vi "NLR3.vi"(8 "X4":dbl, 9 "X3":dbl, 10 "X2":dbl, 11 "X1":dbl) -> (2 "s? t:f":dbl)   [LabVIEW 2013]
uses:
  <vilib>/express/express arith-compare/Formula/XNode/ExpressFormulaBlockNode.xnode
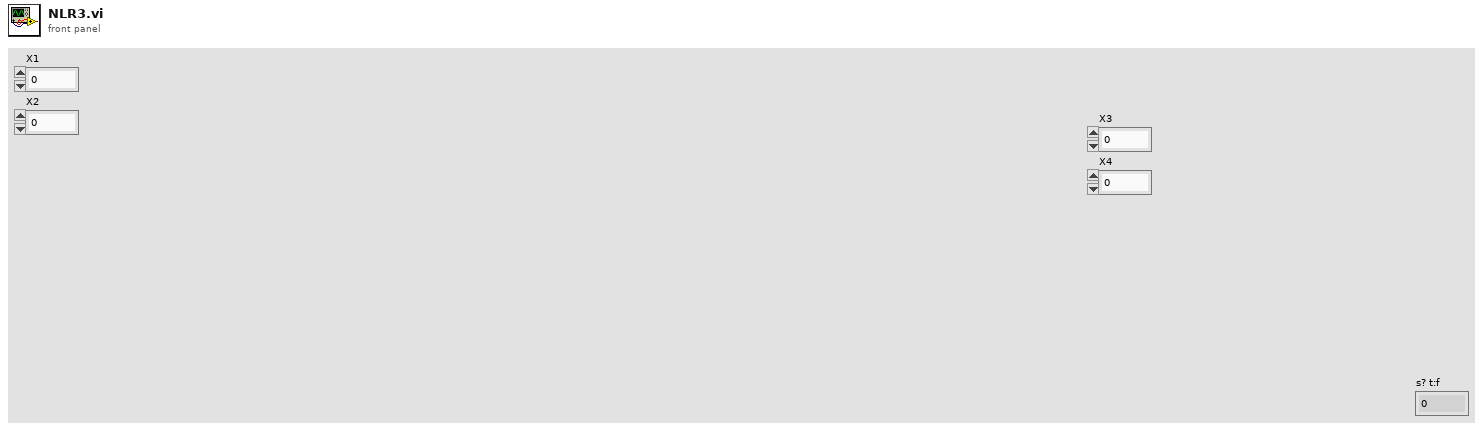
[diagram p1: front panel]
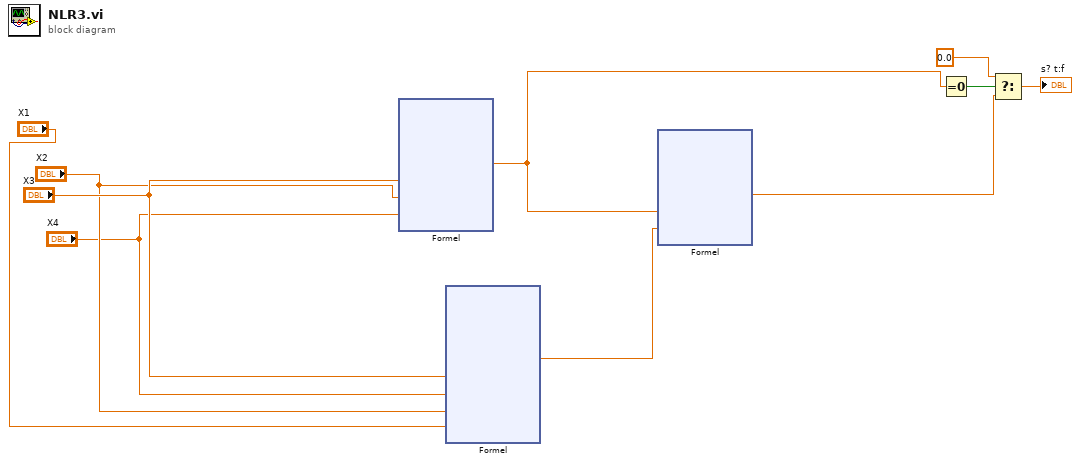
[diagram p0: block diagram]
diagram:
  n1 = xnode "Formel"("X3"="X3", "X2"="X2", "X4"="X4") -> ("Ergebnis"=w5:dbl)  [unwired: 1 in, 1 out]
  n2 = xnode "Formel"("X3"="X3", "X4"="X4", "X2"="X2", "X1"="X1") -> ("Ergebnis"=w6:dbl)  [unwired: 1 in, 1 out]
  n3 = xnode "Formel"("b"=w5, "a"=w6) -> ("Ergebnis"=w7:dbl)  [unwired: 1 in, 1 out]
  n4 = Equal To 0? ("Gleich 0?")(x=w5) -> (x = 0?=w10:bool)
  n5 = Select ("Auswählen")(t=0.0 ("value below threshold 2"), s=w10, f=w7) -> (s? t:f=→"s? t:f":dbl)
